vi "Get Register.vi"(11 "TEMPLATE jettl in":refnum<class "TEMPLATE jettl.lvclass">) -> (2 "Register":refnum<event-registration>)   [LabVIEW 2021, in "_Template.lvlib" / "Templates.lvlib" / "TEMPLATE jettl.lvlib" / "TEMPLATE jettl.lvclass"]
uses:
  TEMPLATE jettl.lvclass
  jettl/jettl/Msg Strategy/Msg Strategy.lvclass
  TEMPLATE jettl.lvclass/TEMPLATE jettl.ctl
  jettl/jettl/jettl/jettl.lvclass
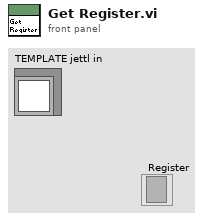
[diagram p1: front panel]
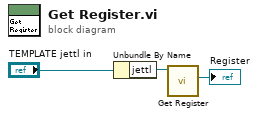
[diagram p0: block diagram]
diagram:
  n1 = Unbundle By Name("TEMPLATE jettl in") -> ("jettl"=w2:refnum<class "jettl.lvclass">)
  n2 = call-dynamic "Get Register.vi"("jettl in"=w2) -> ("Register"=→"Register":refnum<event-registration>)  [unwired: 10 in]
